vi "modify assembly.vi"(8 "error in":errorcluster, 9 "new":T1={"name"="", "Instance ID"=100, "Type"=enum."Producing", "Size (bytes)"=32}, 10 "original":T1={"name"="", "Instance ID"=100, "Type"=enum."Producing", "Size (bytes)"=32}, 11 "EthernetIP configuration in":refnum<class "EthernetIP configuration.lvclass">) -> (0 "error out":errorcluster, 1 "channel classification changed":refnum<class "EthernetIP Channel.lvclass">[](array[class]), 2 "invalidated channels":refnum<class "EthernetIP Channel.lvclass">[](array[class]), 3 "EthernetIP configuration out":refnum<class "EthernetIP configuration.lvclass">)   [LabVIEW 2013, in "EthernetIP configuration.lvclass"]
uses:
  EthernetIP configuration.lvclass
  assembly definition.ctl
  assembly type.ctl
  channel/EthernetIP Channel.lvclass
  EthernetIP configuration.lvclass/EthernetIP configuration.ctl
  channel/EthernetIP Channel.lvclass/EthernetIP Channel.ctl
  <vilib>/NI/Tag Bus Module Framework/channel/TBM channel.lvclass/TBM channel.ctl
  channel/Write Instance ID.vi
  <vilib>/NI/Tag Bus Module Framework/channel/Read channel classification.vi
  <vilib>/NI/Tag Bus Module Framework/channel/Write channel classification.vi
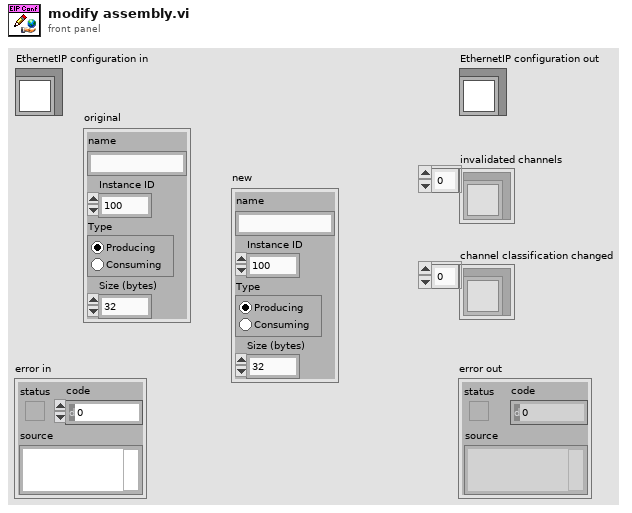
[diagram p1: front panel]
types:
  T1 = typedef "EthernetIP configuration.lvclass/assembly definition.ctl" = cluster{"name":string, "Instance ID":u32, "Type":T2, "Size (bytes)":u32}
  T2 = typedef "EthernetIP configuration.lvclass/assembly type.ctl" = enum32{"Producing", "Consuming"}
  T3 = typedef "TBM channel.lvclass/channel classification.ctl" = enum16{"input data", "output data", "processing parameter", "processing result"}
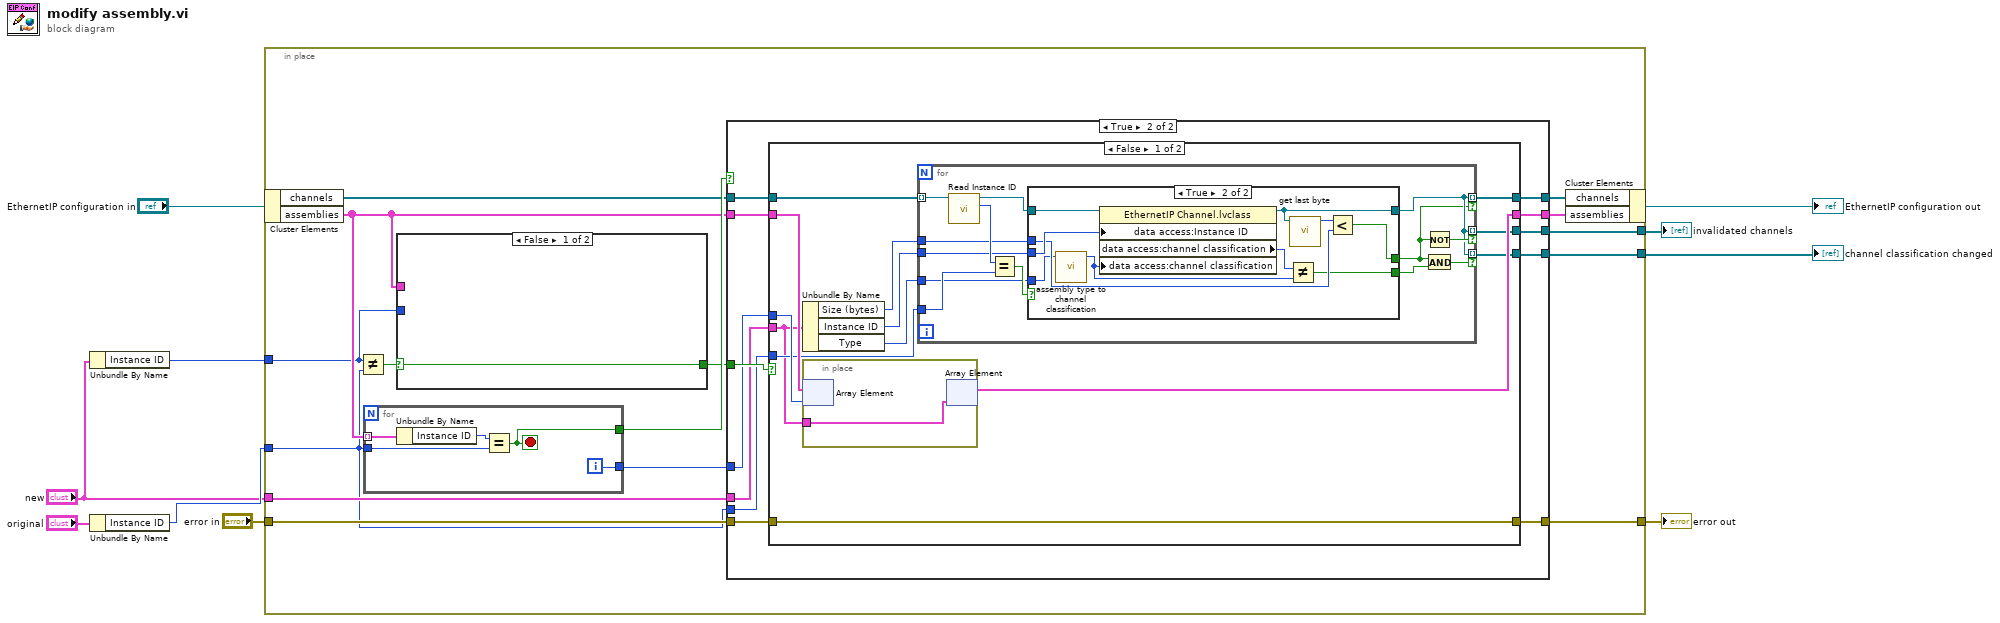
[diagram p0: block diagram]
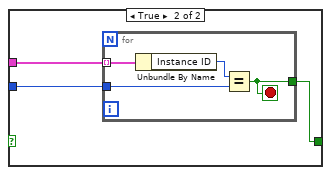
[diagram p2: hidden frame]
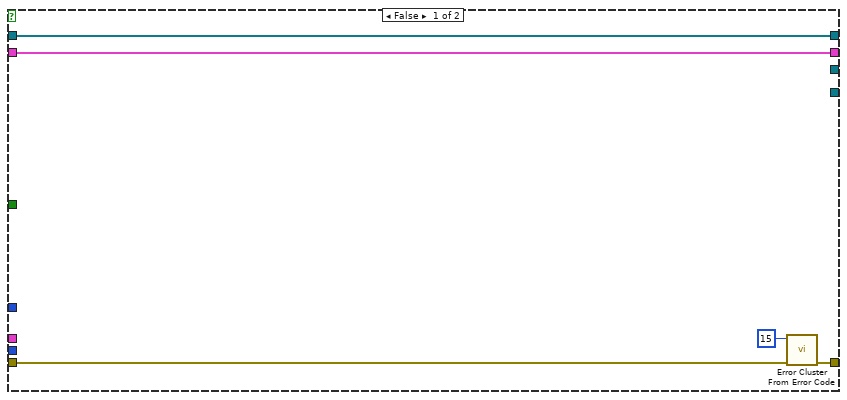
[diagram p3: hidden frame]
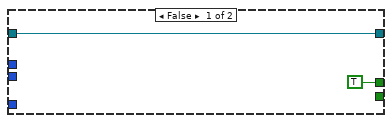
[diagram p4: hidden frame]
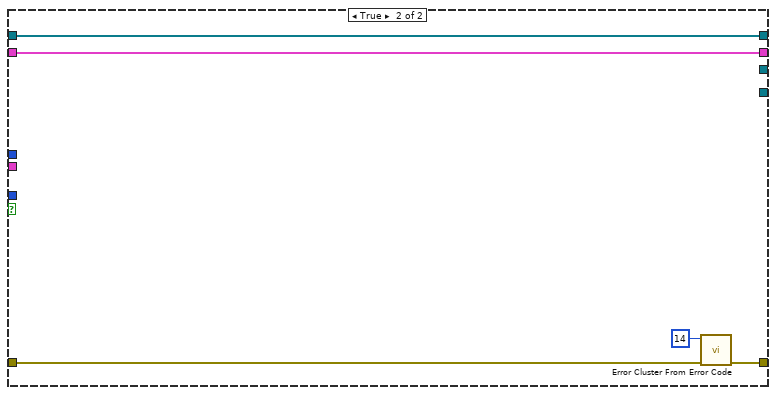
[diagram p5: hidden frame]
diagram:
  n1 = Unbundle By Name("new") -> ("Instance ID"=w6:u32)
  n2 = Unbundle By Name("original") -> ("Instance ID"=w7:u32)
  n3 = in-place {
    in-place-border: w7 -> [w14]
    in-place-border: w6 -> [w13]
    in-place-border: "error in" -> [w20]
    in-place-border: [w19] -> w4
    in-place-border: "new" -> [w16]
    in-place-border: [w15] -> w2
    in-place-border: [w11] -> w1
    n4 = in-place-cluster #1("EthernetIP configuration in") -> ("channels"=w21:refnum<class "EthernetIP Channel.lvclass">[], "assemblies"=w24:T1[])
    n5 = Not Equal?(x=w13, y=w14) -> (x != y?=w12:bool)
    n6 = for {
      tunnel: w24 -> [w99] mode=indexing
      tunnel: [w97] -> w25
      tunnel: [w96] -> w17
      tunnel: w14 -> [w95]
      i -> [w96]
      stop <- w97 stop-if-true
      n7 = Unbundle By Name(w99) -> ("Instance ID"=w98:u32)
      n8 = Equal?(x=w98, y=w95) -> (x = y?=w97:bool)
    }
    n9 = case shown="False" w12 {
      selector: w12 -> [w26 _]
      tunnel: w24 -> [_ w29]
      tunnel: [w26 w28] -> w18
      tunnel: w13 -> [_ w27]
      frame False {
      }
      frame True {
        n10 = for {
          tunnel: w29 -> [w33] mode=indexing
          tunnel: [w31] -> w28
          tunnel: w27 -> [w30]
          stop <- w31 stop-if-true
          n11 = Unbundle By Name(w33) -> ("Instance ID"=w32:u32)
          n12 = Equal?(x=w32, y=w30) -> (x = y?=w31:bool)
        }
      }
    }
    n13 = case shown="True" w25 {
      tunnel: w24 -> [w38 w44]
      tunnel: [w38 w45] -> w23
      tunnel: [w37 w46] -> w22
      tunnel: w21 -> [w37 w47]
      tunnel: w20 -> [w36 w48]
      tunnel: [w34 w49] -> w19
      tunnel: w18 -> [_ w50]
      tunnel: w17 -> [_ w43]
      tunnel: w16 -> [_ w42]
      tunnel: w14 -> [_ w41]
      tunnel: [_ w40] -> w15
      tunnel: [_ w39] -> w11
      frame False {
        n14 = call <vilib>:"Error Cluster From Error Code.vi"("error in (no error)"=w36, "error code (0)"=15) -> ("error out"=w34:errorcluster)  [unwired: 7 in]
      }
      frame True {
        n15 = case shown="False" w50 {
          tunnel: [w60 w93] -> w49
          tunnel: w48 -> [w60 w92]
          tunnel: w47 -> [w55 w91]
          tunnel: [w52 w91] -> w46
          tunnel: [w61 w90] -> w45
          tunnel: w44 -> [w63 w90]
          tunnel: w43 -> [w62 _]
          tunnel: w42 -> [w58 _]
          tunnel: w41 -> [w59 _]
          tunnel: [w56 _] -> w40
          tunnel: [w51 _] -> w39
          frame False {
            n16 = Unbundle By Name(w58) -> ("Size (bytes)"=w54:u32, "Instance ID"=w57:u32, "Type"=w53:T2)
            n17 = in-place {
              in-place-border: w58 -> [w89]
              n18 = in-place-array #2(w63, w62) -> ()  [unwired: 1 out]
              n19 = in-place-array #2(w89) -> (w61:T1[])  [unwired: 1 out]
            }
            n20 = for {
              tunnel: w55 -> [w76] mode=indexing
              tunnel: w59 -> [w74]
              tunnel: [w67] -> w52 mode=indexing if=w66
              tunnel: w57 -> [w71]
              tunnel: [w67] -> w56 mode=indexing if=w70
              tunnel: w54 -> [w69]
              tunnel: w53 -> [w68]
              tunnel: [w67] -> w51 mode=indexing if=w64
              n21 = call "Read Instance ID.vi"("EthernetIP Channel in"=w76) -> ("Instance ID"=w75:u32, "EthernetIP Channel out"=w73:refnum<class "EthernetIP Channel.lvclass">)  [unwired: 8 in, 1 out]
              n22 = Equal?(x=w75, y=w74) -> (x = y?=w72:bool)
              n23 = case shown="True" w72 {
                tunnel: w73 -> [w77 w88]
                tunnel: [w77 w87] -> w67
                tunnel: w71 -> [_ w86]
                tunnel: [TRUE w83] -> w66
                tunnel: w69 -> [_ w84]
                tunnel: w68 -> [_ w82]
                tunnel: [_ w79] -> w65
                frame False {
                }
                frame True {
                  n24 = call "assembly type to channel classification.vi"("Type"=w82) -> ("channel classification"=w80:T3)  [unwired: 10 in]
                  n25 = property class="EthernetIP Channel.lvclass"(reference=w88, "data access:Instance ID"=w86, "data access:channel classification"=w80) -> (reference out=w87:refnum<class "EthernetIP Channel.lvclass">, "data access:channel classification"=w81:T3)  [unwired: 1 in, 1 out]
                  n26 = Not Equal?(x=w81, y=w80) -> (x != y?=w79:bool)
                  n27 = call "get last byte.vi"("EthernetIP Channel in"=w87) -> ("last byte"=w85:i32)  [unwired: 10 in]
                  n28 = Less?(x=w85, y=w84) -> (x < y?=w83:bool)
                }
              }
              n29 = Not(x=w66) -> (.not. x?=w70:bool)
              n30 = And(x=w66, y=w65) -> (x .and. y?=w64:bool)
            }
          }
          frame True {
            n31 = call <vilib>:"Error Cluster From Error Code.vi"("error in (no error)"=w92, "error code (0)"=14) -> ("error out"=w93:errorcluster)  [unwired: 7 in]
          }
        }
      }
    }
    n32 = in-place-cluster #1("channels"=w22, "assemblies"=w23) -> (→"EthernetIP configuration out":refnum<class "EthernetIP configuration.lvclass">)
  }
  "error out" <- w4
  "invalidated channels" <- w2
  "channel classification changed" <- w1
